vi "Filter Graves.vi"(8 "Error In":errorcluster, 11 "GObjects":refnum<vi>[](array[refnum])) -> (0 "Error Out":errorcluster, 3 "Graves":refnum<vi>[](array[refnum]))   [LabVIEW 2017, in "Toolkit.lvlib"]
doc: "Filters an array of GObject references and keeps only references to graves. Any references that are NOT to a grave are closed. A grave is a Diagram Disable Structure with a RIP bookmark tag for its label, a.ka. tombstone."
uses:
  Toolkit.lvlib
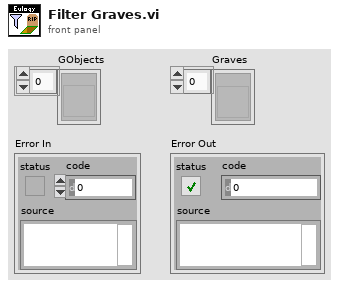
[diagram p1: front panel]
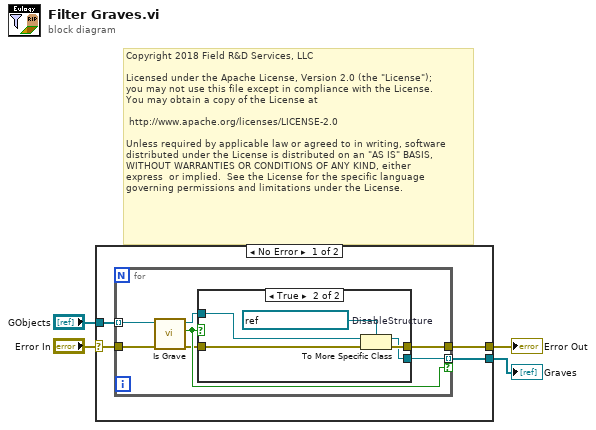
[diagram p0: block diagram]
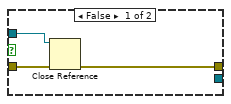
[diagram p2: hidden frame]
diagram:
  # "Copyright 2018 Field R&D Services, LLC\n\nLicensed under the Apache License, Version 2.0 (the \"License\");\nyou may not use this file except in compliance with the License.\nYou may obtain a copy of the License at\n\n\thttp://www.apache.org/licenses/LICENSE-2.0\n\nUnless required by applicable law or agreed to in writing, software\ndistributed under the License is distributed on an \"AS IS\" BASIS,\nWITHOUT WARRANTIES OR CONDITIONS OF ANY KIND, either \nexpress  or implied.  See the License for the specific language \ngoverning permissions and limitations under the License."
  n1 = case shown="No Error" "Error In" {
    selector: "Error In" -> [w5 w24]
    tunnel: [w8 w24] -> w4
    tunnel: [w7 _] -> w3
    tunnel: "GObjects" -> [w6 _]
    frame No Error {
      n2 = for {
        tunnel: [w11] -> w7 mode=indexing if=w14
        tunnel: [w12] -> w8
        tunnel: w6 -> [w10] mode=indexing
        tunnel: w5 -> [w9]
        n3 = call "Is Grave.vi"("Error In"=w9, "GObject In"=w10) -> ("Error Out"=w13:errorcluster, "Grave?"=w14:bool, "GObject Out"=w15:refnum<vi>)  [unwired: 7 in]
        n4 = case shown="True" w14 {
          tunnel: w15 -> [w18 w23]
          tunnel: w13 -> [w17 w22]
          tunnel: [w16 w20] -> w12
          tunnel: [_ w19] -> w11
          frame False {
            n5 = Close Reference(reference=w18, error in (no error)=w17) -> (error out=w16:errorcluster)
          }
          frame True {
            w21 = refnum<vi> refnum  # DisableStructure
            n6 = To More Specific Class(target class=w21, reference=w23, error in=w22) -> (specific class reference=w19:refnum<vi>, error out=w20:errorcluster)
          }
        }
      }
    }
    frame Error {
    }
  }
  "Error Out" <- w4
  "Graves" <- w3
